vi "Configure Limit Test Result Pattern.vi"(0 "VISA resource name":refnum<visa-resource-name>, 1 "Limit Test Pass Pattern (16383)":i32=16383, 2 "Limit Test Upper Exceeding Pattern (16383)":i32=16383, 5 "Channel (0: Channel 1)":i32(ring) items=["Channel 1", "Channel 2"], 7 "Limit Test Number (1)":i32=1, 11 "error in (no error)":errorcluster, 12 "Limit Test Failure Pattern (16383 16838)":i32=16383, 13 "Limit Test Lower Exceeding Pattern (16383)":i32=16383) -> (4 "VISA resource name out":refnum<visa-resource-name>, 15 "error out":errorcluster)   [LabVIEW 2023, in "Agilent B2900 Series.lvlib"]
doc: "Defines bit patterns used to indicate different limit test results. \n\n<B>Note:</B>\nThis VI is not applicable for Agilent models B2961A, B2962A, B2961B, B2962B, B2961C and B2962C."
uses:
  Agilent B2900 Series.lvlib
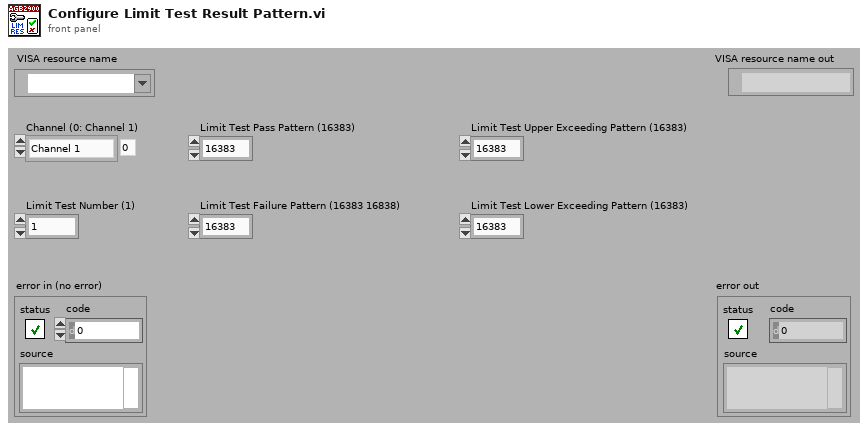
[diagram p1: front panel]
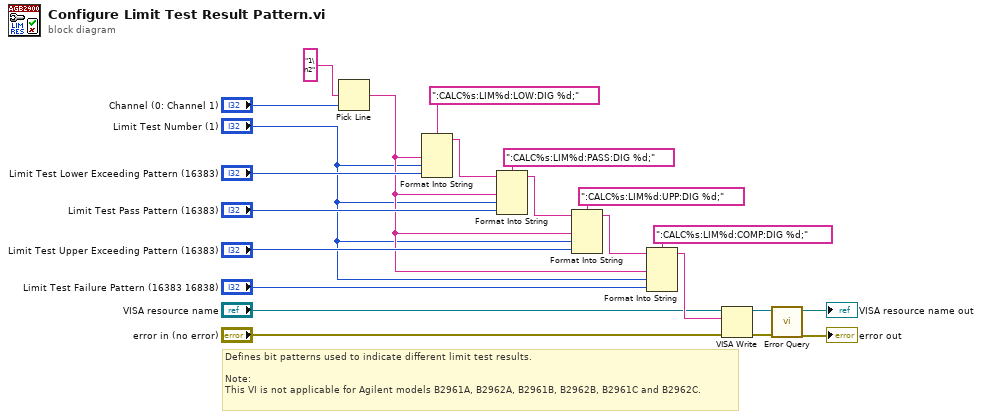
[diagram p0: block diagram]
diagram:
  # "Defines bit patterns used to indicate different limit test results. \n\nNote:\nThis VI is not applicable for Agilent models B2961A, B2962A, B2961B, B2962B, B2961C and B2962C."
  n1 = Pick Line(multi-line string="1\n2" ("string (\"\")"), line index="Channel (0: Channel 1)") -> (output string=w3:string)  [unwired: 1 in]
  n2 = Format Into String(format string=":CALC%s:LIM%d:LOW:DIG %d;", w3, "Limit Test Number (1)", "Limit Test Lower Exceeding Pattern (16383)") -> (resulting string=w21:string)  [unwired: 2 in, 1 out]
  n3 = Format Into String(format string=":CALC%s:LIM%d:PASS:DIG %d;", initial string=w21, w3, "Limit Test Number (1)", "Limit Test Pass Pattern (16383)") -> (resulting string=w19:string)  [unwired: 1 in, 1 out]
  n4 = Format Into String(format string=":CALC%s:LIM%d:UPP:DIG %d;", initial string=w19, w3, "Limit Test Number (1)", "Limit Test Upper Exceeding Pattern (16383)") -> (resulting string=w17:string)  [unwired: 1 in, 1 out]
  n5 = Format Into String(format string=":CALC%s:LIM%d:COMP:DIG %d;", initial string=w17, w3, "Limit Test Number (1)", "Limit Test Failure Pattern (16383 16838)") -> (resulting string=w15:string)  [unwired: 1 in, 1 out]
  n6 = VISA Write(VISA resource name="VISA resource name", write buffer=w15, error in (no error)="error in (no error)") -> (VISA resource name out=w12:refnum<visa-resource-name>, error out=w11:errorcluster)  [unwired: 1 out]
  n7 = call "Error Query.vi"("error in (no error)"=w11, "VISA resource name"=w12) -> ("error out"=→"error out":errorcluster, "VISA resource name out"=→"VISA resource name out":refnum<visa-resource-name>)  [unwired: 6 in, 2 out]
